vi "mux10-1_chan7.vi"(8 "error in":errorcluster) -> (0 "error out":errorcluster)   [LabVIEW 2018, in "MB switches Module.lvlib"]
doc: "_____\nCreated using DQMH Event Scripter 6.0.0.122."
uses:
  MB switches Module.lvlib
  mux10-1_chan7 Argument--cluster.ctl
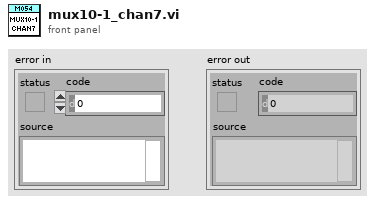
[diagram p1: front panel]
types:
  T1 = typedef "MB switches Module.lvlib/mux10-1_chan7 Argument--cluster.ctl" = cluster{"Boolean":bool}
  T2 = typedef "MB switches Module.lvlib/Request Events--cluster.ctl" = cluster{"Stop Module":refnum<user-event>, "Do Something Else and Wait for Reply":refnum<user-event>, "Show Panel":refnum<user-event>, "Hide Panel":refnum<user-event>, "Get Module Execution Status":refnum<user-event>, "Show Diagram":refnum<user-event>, "inst.Counter":refnum<user-event>, "inst.Open":refnum<user-event>, "inst.Close":refnum<user-event>, "inst.Optos":refnum<user-event>, "mux10-1_chan0":refnum<user-event>, "mux6-1_chan0":refnum<user-event>, "DMM I 0.5_10":refnum<user-event>, "mux10-1_chan1":refnum<user-event>, "mux10-1_chan2":refnum<user-event>, "mux10-1_chan3":refnum<user-event>, "mux10-1_chan4":refnum<user-event>, "mux10-1_chan5":refnum<user-event>, "mux10-1_chan6":refnum<user-event>, "mux10-1_chan7":refnum<user-event>, "mux10-1_chan8":refnum<user-event>, "mux10-1_chan9":refnum<user-event>, "mux10-1_chan10":refnum<user-event>, "mux6-1_chan1_1":refnum<user-event>, "mux6-1_chan1_2":refnum<user-event>, "mux6-1_chan2_1":refnum<user-event>, "mux6-1_chan2_2":refnum<user-event>}
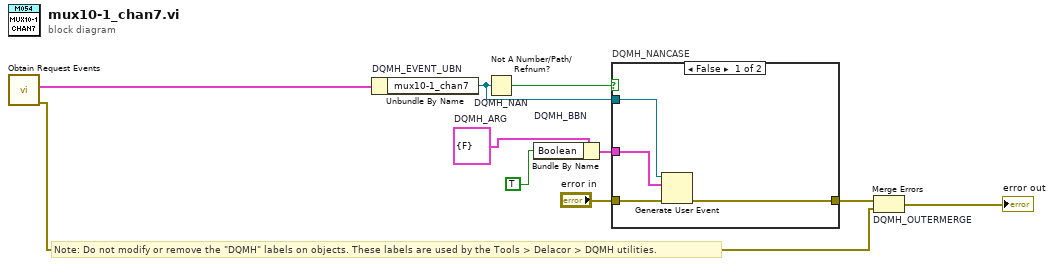
[diagram p0: block diagram]
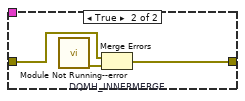
[diagram p2: hidden frame]
diagram:
  w4 = T1 {"Boolean"=FALSE}  # DQMH_ARG
  # "Note: Do not modify or remove the \"DQMH\" labels on objects. These labels are used by the Tools > Delacor > DQMH utilities."
  n1 = call "Obtain Request Events.vi"() -> ("error out"=w2:errorcluster, "Switches Module Request Events"=w1:T2)  [unwired: 10 in]
  n2 = Unbundle By Name "DQMH_EVENT_UBN"(w1) -> ("mux10-1_chan7"=w6:refnum<user-event>)
  n3 = Not A Number/Path/Refnum? "DQMH_NAN"(number/path/refnum=w6) -> (NaN/Path/Refnum?=w7:bool)
  n4 = Bundle By Name "DQMH_BBN"(cluster=w4, "Boolean"=TRUE) -> (w8:T1)
  n5 = case "DQMH_NANCASE" shown="False" w7 {
    tunnel: "error in" -> [w14 w17]
    tunnel: [w13 w16] -> w5
    tunnel: w6 -> [w12 _]
    tunnel: w8 -> [w11 _]
    frame False {
      n6 = Generate User Event(user event=w12, event data cluster=w11, error in=w14) -> (error out=w13:errorcluster)  [unwired: 1 in, 1 out]
    }
    frame True {
      n7 = call "Module Not Running--error.vi"() -> ("error out"=w15:errorcluster)  [unwired: 11 in]
      n8 = Merge Errors "DQMH_INNERMERGE"(w17, w15) -> (w16:errorcluster)
    }
  }
  n9 = Merge Errors "DQMH_OUTERMERGE"(w5, w2) -> (→"error out":errorcluster)
